vi "User_Database_Change_Password_Confirm.vi"(8 "error in (no error)":errorcluster caption="Error In") -> (0 "error out":errorcluster caption="Error Out", 2 "User_Right":i32, 3 "OK":bool)   [LabVIEW 2020]
uses:
  <vilib>/Utility/error.llb/whitespace.ctl
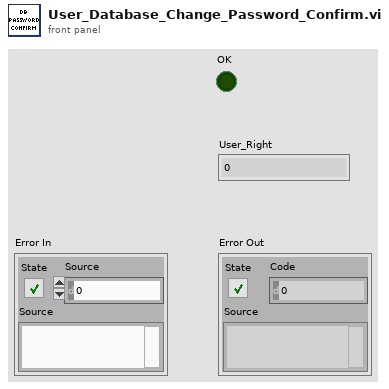
[diagram p1: front panel]
types:
  T1 = typedef "whitespace.ctl" = u16
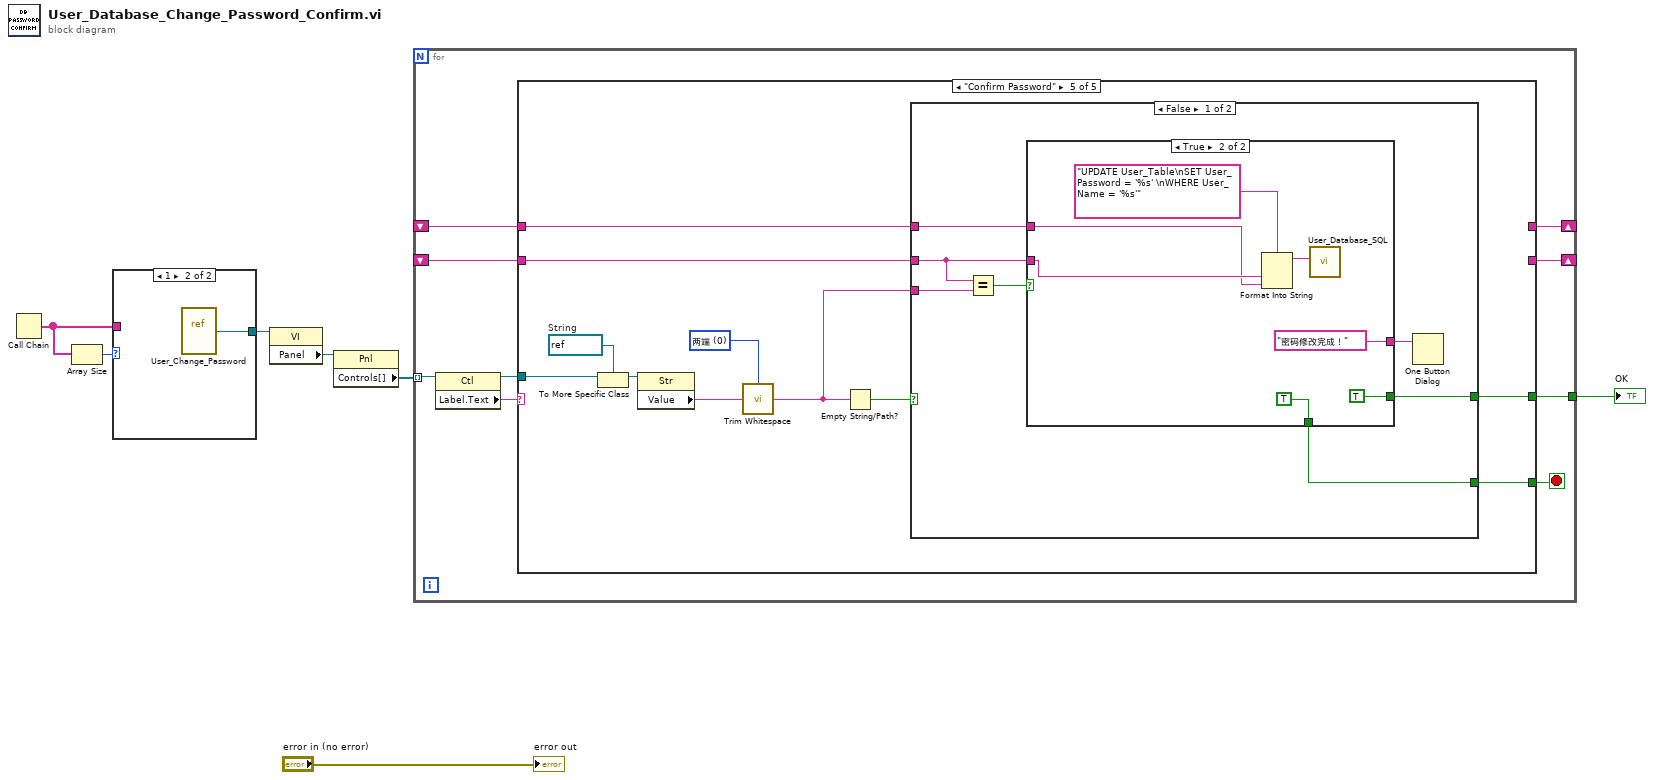
[diagram p0: block diagram]
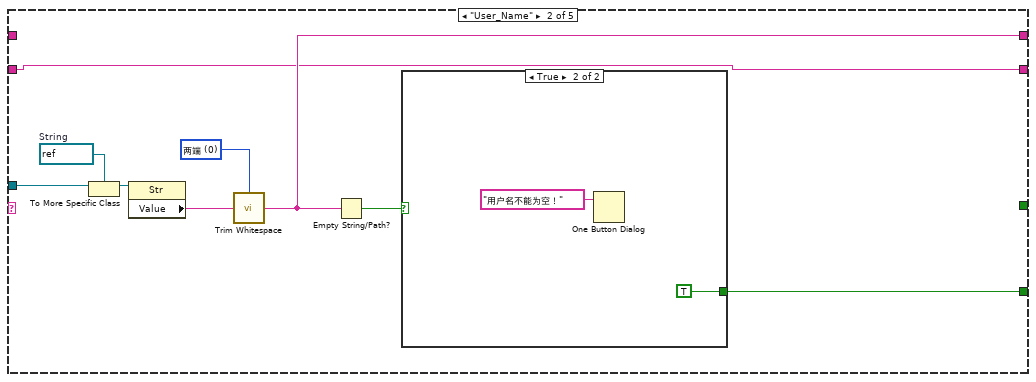
[diagram p3: hidden frame]
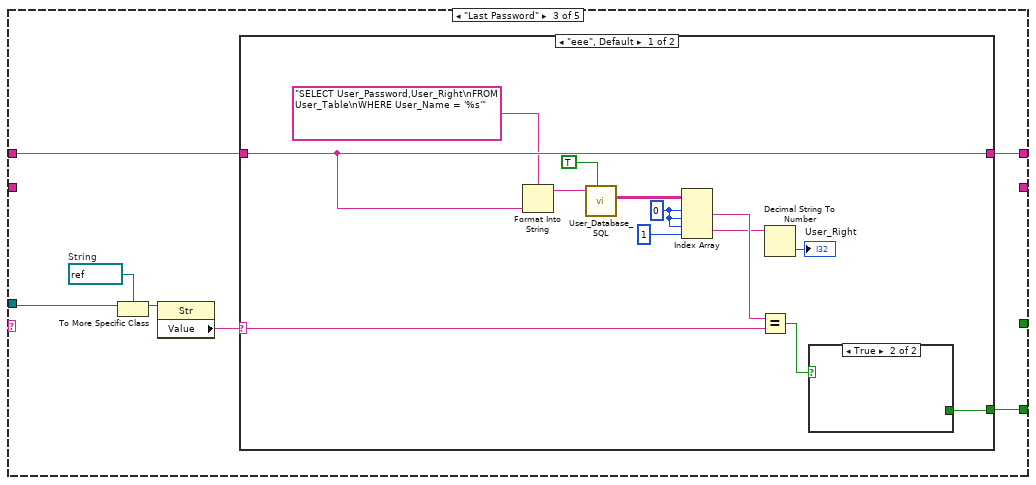
[diagram p5: hidden frame]
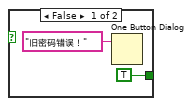
[diagram p6: hidden frame]
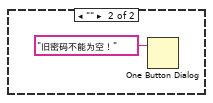
[diagram p7: hidden frame]
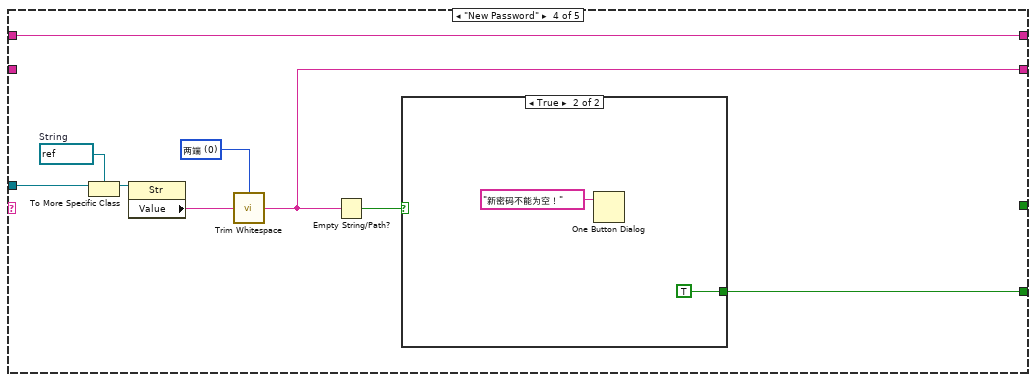
[diagram p8: hidden frame]
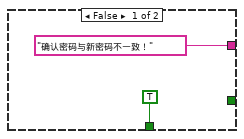
[diagram p10: hidden frame]
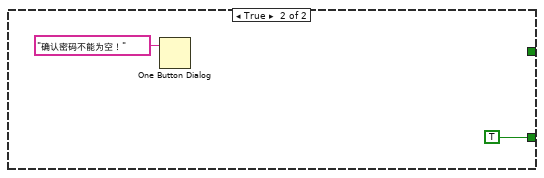
[diagram p11: hidden frame]
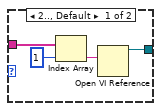
[diagram p12: hidden frame]
diagram:
  n1 = Call Chain() -> (call chain=w4:string[])
  n2 = Array Size(array=w4) -> (size(s)=w5:i32)
  n3 = case shown="1" w5 {
    tunnel: [w9 w12] -> w2
    tunnel: w4 -> [w8 _]
    frame 2.., Default {
      n4 = Index Array(array=w8, index=1 ("索引")) -> (element=w10:string)
      n5 = Open VI Reference(vi path=w10) -> (vi reference=w9:refnum<vi>)  [unwired: 5 in, 1 out]
    }
    frame 1 {
      n6 = vi-ref "User_Change_Password.vi"() -> (w12:refnum<vi>)
    }
  }
  n7 = property class="VI"(reference=w2) -> ("Panel"=w3:refnum<vi>)  [unwired: 1 in, 2 out]
  n8 = property class="Pnl"(reference=w3) -> ("Controls[]"=w6:refnum<vi>[])  [unwired: 1 in, 2 out]
  n9 = for {
    tunnel: w6 -> [w21] mode=indexing
    shift-right: [w18] -> _
    shift-left: _ -> [w17]
    tunnel: [w16] -> w1
    shift-right: [w14] -> _
    shift-left: _ -> [w13]
    stop <- w19 stop-if-true
    n10 = property class="Ctl"(reference=w21) -> (reference out=w20:refnum<vi>, "Label.Text"=w15:string)  [unwired: 1 in, 1 out]
    n11 = case shown="\"Confirm Password\"" w15 {
      tunnel: w20 -> [_ w31 w38 w65 w78]
      tunnel: [_ w26 w34 w60 w73] -> w19
      tunnel: [w22 w24 w35 w57 _] -> w18
      tunnel: w17 -> [w22 _ w37 w57 w68]
      tunnel: [_ _ _ _ w70] -> w16
      tunnel: [_ w23 _ w58 _] -> w14
      tunnel: w13 -> [_ w23 _ _ w69]
      frame "eee", Default {
      }
      frame "User_Name" {
        w28 = T1 0 items=["两端", "字符串首端", "字符串末端"] ("location (both)")
        w30 = refnum<vi> refnum  # String
        n12 = To More Specific Class(target class=w30, reference=w31) -> (specific class reference=w29:refnum<vi>)  [unwired: 1 in, 1 out]
        n13 = property class="Str"(reference=w29) -> ("Value"=w25:string)  [unwired: 1 in, 2 out]
        n14 = call <vilib>:"Trim Whitespace.vi"("string"=w25, "location (both)"=w28) -> ("trimmed string"=w24:string)
        n15 = Empty String/Path?(string/path=w24) -> (empty?=w27:bool)
        n16 = case shown="True" w27 {
          tunnel: [_ TRUE] -> w26
          frame False {
          }
          frame True {
            n17 = One Button Dialog(message="用户名不能为空！" ("消息")) -> ()  [unwired: 1 in, 1 out]
          }
        }
      }
      frame "Last Password" {
        w40 = refnum<vi> refnum  # String
        n18 = To More Specific Class(target class=w40, reference=w38) -> (specific class reference=w39:refnum<vi>)  [unwired: 1 in, 1 out]
        n19 = property class="Str"(reference=w39) -> ("Value"=w36:string)  [unwired: 1 in, 2 out]
        n20 = case shown="\"eee\", Default" w36 {
          selector: w36 -> [w53 _]
          tunnel: w37 -> [w52 _]
          tunnel: [w52 _] -> w35
          tunnel: [w42 _] -> w34
          frame "eee", Default {
            w46 = 0 ("索引 (行)")
            n21 = Format Into String(format string="SELECT User_Password,User_Right\nFROM User_Table\nWHERE User_Name = '%s'" ("SQL query"), w52) -> (resulting string=w50:string)  [unwired: 2 in, 1 out]
            n22 = call "User_Database_SQL.vi"("Get Record"=TRUE, "SQL query"=w50) -> ("Record"=w48:string[][])  [unwired: 7 in, 2 out]
            n23 = Index Array(array=w48, index (row) #1=w46, index (col) #1=w46, index (row) #2=w46, index (col) #2=1 ("禁用的索引 (列)")) -> (element #1=w47:string, element #2=w44:string)
            n24 = Equal?(x=w47, y=w53) -> (x = y?=w43:bool)
            n25 = Decimal String To Number(string=w44) -> (number=→"User_Right":i32)  [unwired: 2 in, 1 out]
            n26 = case shown="True" w43 {
              tunnel: [TRUE _] -> w42
              frame False {
                n27 = One Button Dialog(message="旧密码错误！" ("消息")) -> ()  [unwired: 1 in, 1 out]
              }
              frame True {
              }
            }
          }
          frame "" {
            n28 = One Button Dialog(message="旧密码不能为空！" ("消息")) -> ()  [unwired: 1 in, 1 out]
          }
        }
      }
      frame "New Password" {
        w62 = T1 0 items=["两端", "字符串首端", "字符串末端"] ("location (both)")
        w64 = refnum<vi> refnum  # String
        n29 = To More Specific Class(target class=w64, reference=w65) -> (specific class reference=w63:refnum<vi>)  [unwired: 1 in, 1 out]
        n30 = property class="Str"(reference=w63) -> ("Value"=w59:string)  [unwired: 1 in, 2 out]
        n31 = call <vilib>:"Trim Whitespace.vi"("string"=w59, "location (both)"=w62) -> ("trimmed string"=w58:string)
        n32 = Empty String/Path?(string/path=w58) -> (empty?=w61:bool)
        n33 = case shown="True" w61 {
          tunnel: [_ TRUE] -> w60
          frame False {
          }
          frame True {
            n34 = One Button Dialog(message="新密码不能为空！" ("消息")) -> ()  [unwired: 1 in, 1 out]
          }
        }
      }
      frame "Confirm Password" {
        w75 = T1 0 items=["两端", "字符串首端", "字符串末端"] ("location (both)")
        w77 = refnum<vi> refnum  # String
        n35 = To More Specific Class(target class=w77, reference=w78) -> (specific class reference=w76:refnum<vi>)  [unwired: 1 in, 1 out]
        n36 = property class="Str"(reference=w76) -> ("Value"=w72:string)  [unwired: 1 in, 2 out]
        n37 = call <vilib>:"Trim Whitespace.vi"("string"=w72, "location (both)"=w75) -> ("trimmed string"=w71:string)
        n38 = Empty String/Path?(string/path=w71) -> (empty?=w74:bool)
        n39 = case shown="False" w74 {
          tunnel: [w83 TRUE] -> w73
          tunnel: w71 -> [w85 _]
          tunnel: [w82 _] -> w70
          tunnel: w69 -> [w81 _]
          tunnel: w68 -> [w80 _]
          frame False {
            n40 = Equal?(x=w81, y=w85) -> (x = y?=w84:bool)
            n41 = case shown="True" w84 {
              tunnel: [TRUE TRUE] -> w83
              tunnel: [_ TRUE] -> w82
              tunnel: w81 -> [_ w90]
              tunnel: w80 -> [_ w89]
              tunnel: ["确认密码与新密码不一致！" ("消息") "密码修改完成！" ("消息")] -> w79
              frame False {
              }
              frame True {
                n42 = Format Into String(format string="UPDATE User_Table\nSET User_Password = '%s' \nWHERE User_Name = '%s'" ("SQL query"), w90, w89) -> (resulting string=w92:string)  [unwired: 2 in, 1 out]
                n43 = call "User_Database_SQL.vi"("SQL query"=w92) -> ()  [unwired: 8 in, 3 out]
              }
            }
            n44 = One Button Dialog(message=w79) -> ()  [unwired: 1 in, 1 out]
          }
          frame True {
            n45 = One Button Dialog(message="确认密码不能为空！" ("消息")) -> ()  [unwired: 1 in, 1 out]
          }
        }
      }
    }
  }
  "OK" <- w1
  "error out" <- "error in (no error)"
